vi "CSMSVMgr unload File.vi"(8 "error in (no error)":errorcluster, 10 "Path":path, 11 "CSM-Static-Variable-Manager in":refnum<class "CSM-Static-Variable-Manager.lvclass">) -> (0 "error out":errorcluster, 3 "CSM-Static-Variable-Manager out":refnum<class "CSM-Static-Variable-Manager.lvclass">)   [LabVIEW 2017, in "INI-Static-Variable-Support.lvlib" / "CSM-Static-Variable-Manager.lvclass"]
uses:
  CSM-Static-Variable-Manager.lvclass
  CSM-Static-Variable-Manager.lvclass/CSM-Static-Variable-Manager.ctl
  LabVIEW-Config/Config.ctl
  LabVIEW-Config/LineToken.ctl
  LabVIEW-Config/LabVIEW-Config.lvlib
  <userlib>/_NEVSTOP/Communicable State Machine(CSM)/Communicable State Machine.lvlib
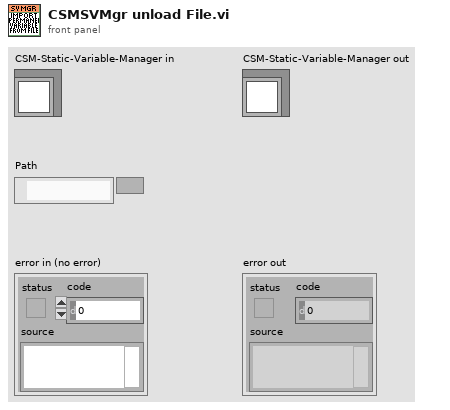
[diagram p1: front panel]
types:
  T1 = typedef "LabVIEW-Config.lvlib/Config.ctl" = cluster{"Path":path, "Lines":string[], "Tokens":T2[], "Modified?":bool}
  T2 = typedef "LabVIEW-Config.lvlib/LineToken.ctl" = enum8{"comment", "section", "key", "more"}
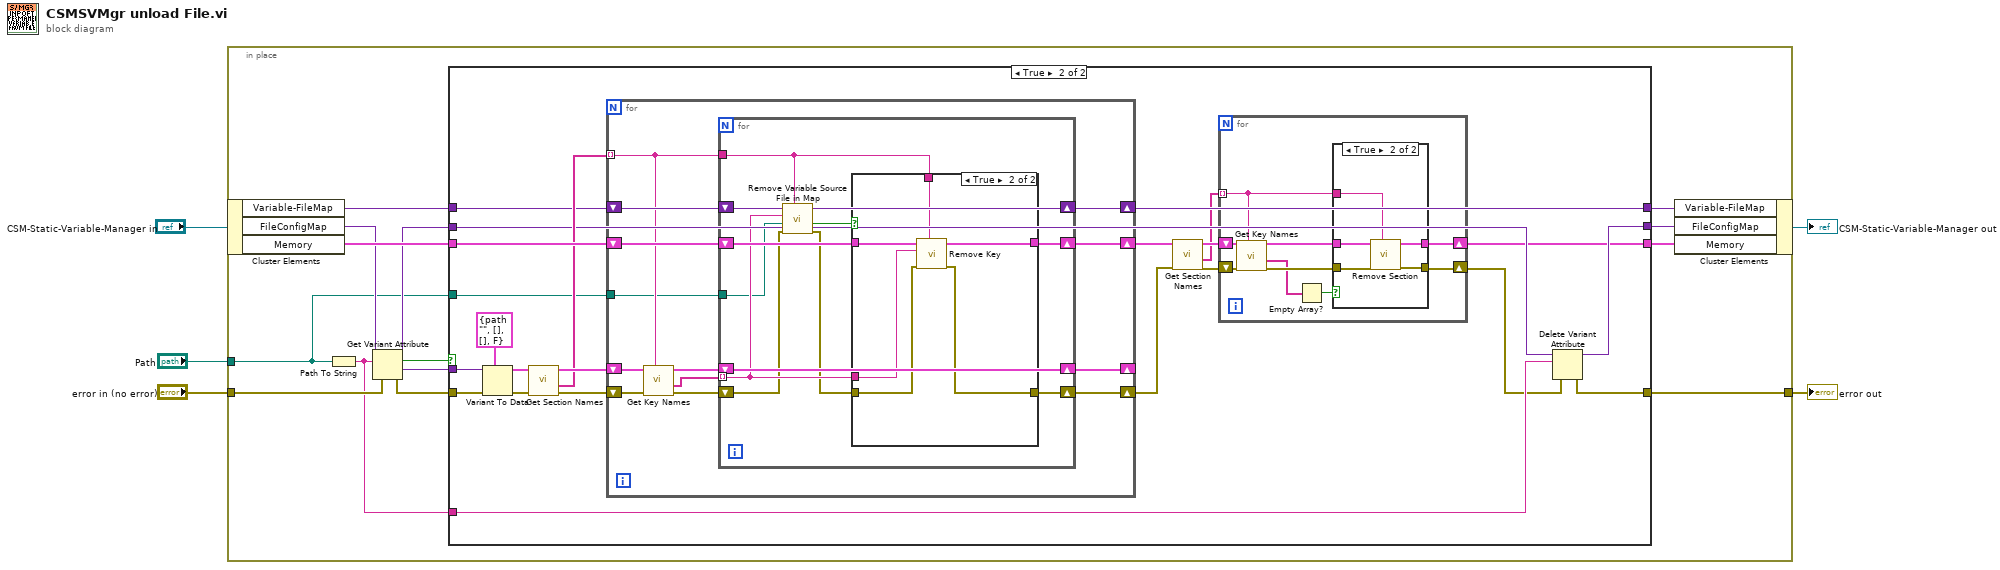
[diagram p0: block diagram]
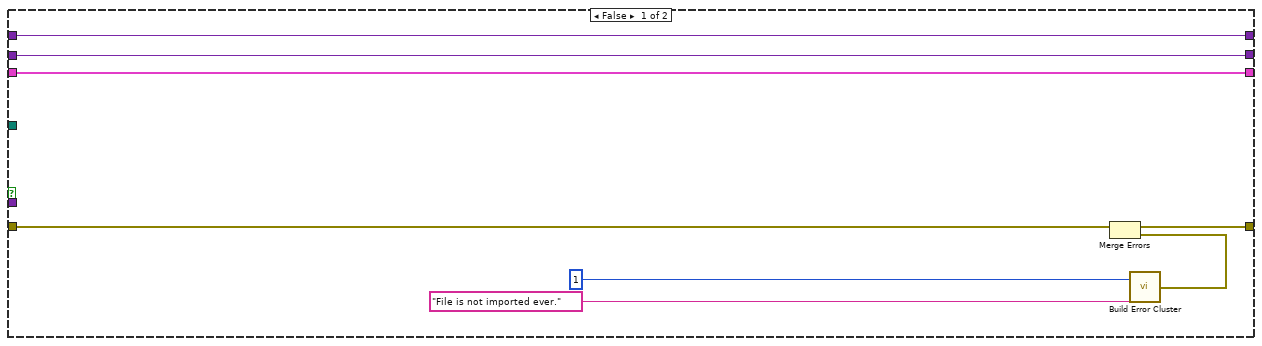
[diagram p2: hidden frame]
diagram:
  n1 = in-place {
    in-place-border: "error in (no error)" -> [w14]
    in-place-border: [w13] -> w2
    in-place-border: "Path" -> [w6]
    n2 = in-place-cluster #1("CSM-Static-Variable-Manager in") -> ("Variable-FileMap"=w9:variant, "FileConfigMap"=w17:variant, "Memory"=w19:T1)
    n3 = Path To String(path=w6) -> (string=w7:string)
    n4 = Get Variant Attribute(Variant=w17, name=w7, error in=w14) -> (duplicate Variant=w12:variant, found=w10:bool, value=w16:variant, error out=w15:errorcluster)  [unwired: 1 in]
    n5 = case shown="True" w10 {
      tunnel: w19 -> [w26 w50]
      tunnel: [w26 w31] -> w18
      tunnel: w16 -> [_ w49]
      tunnel: w15 -> [w25 w48]
      tunnel: [w24 w44] -> w13
      tunnel: w12 -> [w27 w39]
      tunnel: [w27 w43] -> w11
      tunnel: w9 -> [w20 w37]
      tunnel: [w20 w36] -> w8
      tunnel: w7 -> [_ w38]
      tunnel: w6 -> [_ w35]
      frame False {
        n6 = call <userlib>:"Build Error Cluster.vi"("String to Prepend to source (\"\")"="File is not imported ever." ("String to Prepend to source (\"\")"), "code"=1) -> ("error out"=w23:errorcluster)
        n7 = Merge Errors(w25, w23) -> (w24:errorcluster)
      }
      frame True {
        n8 = Variant To Data(error in=w48, type=T1 {"Path"=path "", "Lines"=[], "Tokens"=[], "Modified?"=FALSE}, Variant=w49) -> (data=w45:T1, error out=w47:errorcluster)
        n9 = call "Get Section Names.vi"("error in (no error)"=w47, "Config in"=w45) -> ("error out"=w41:errorcluster, "Section Names"=w40:string[], "Config out"=w42:T1)  [unwired: 7 in]
        n10 = for {
          shift-right: [w76] -> w32
          shift-left: w50 -> [w77]
          shift-right: [w75] -> w30
          shift-left: w41 -> [w73]
          tunnel: w40 -> [w69] mode=indexing
          shift-right: [w72] -> _
          shift-left: w42 -> [w74]
          shift-right: [w71] -> w36
          shift-left: w37 -> [w70]
          tunnel: w35 -> [w67]
          n11 = call "Get Key Names.vi"("Section Name"=w69, "error in (no error)"=w73, "Config in"=w74) -> ("error out"=w68:errorcluster, "Key Names"=w78:string[], "Config out"=w79:T1)  [unwired: 5 in, 1 out]
          n12 = for {
            tunnel: w69 -> [w85]
            tunnel: w78 -> [w84] mode=indexing
            shift-right: [w88] -> w75
            shift-left: w68 -> [w83]
            shift-right: [w91] -> w76
            shift-left: w77 -> [w90]
            shift-right: [w89] -> w72
            shift-left: w79 -> [w89]
            shift-right: [w86] -> w71
            shift-left: w70 -> [w87]
            tunnel: w67 -> [w81]
            n13 = call "Remove Variable Source File in Map.vi"("String"=w85, "error in (no error)"=w83, "dup path"=w81, "Content"=w84, "Variable-FileMap"=w87) -> ("error out"=w82:errorcluster, "No Source Any More?"=w80:bool, "Variant"=w86:variant)  [unwired: 4 in]
            n14 = case shown="True" w80 {
              tunnel: [w93 w99] -> w91
              tunnel: w90 -> [w93 w98]
              tunnel: [w92 w97] -> w88
              tunnel: w85 -> [_ w96]
              tunnel: w84 -> [_ w95]
              tunnel: w82 -> [w92 w94]
              frame False {
              }
              frame True {
                n15 = call "Remove Key.vi"("Section Name"=w96, "error in (no error)"=w94, "Key Name"=w95, "Config in"=w98) -> ("error out"=w97:errorcluster, "Config out"=w99:T1)  [unwired: 5 in, 1 out]
              }
            }
          }
        }
        n16 = call "Get Section Names.vi"("error in (no error)"=w30, "Config in"=w32) -> ("error out"=w33:errorcluster, "Section Names"=w28:string[], "Config out"=w34:T1)  [unwired: 7 in]
        n17 = for {
          shift-right: [w53] -> w31
          shift-left: w34 -> [w59]
          shift-right: [w52] -> w29
          shift-left: w33 -> [w56]
          tunnel: w28 -> [w51] mode=indexing
          n18 = call "Get Key Names.vi"("Section Name"=w51, "error in (no error)"=w56, "Config in"=w59) -> ("error out"=w57:errorcluster, "Key Names"=w55:string[], "Config out"=w58:T1)  [unwired: 5 in, 1 out]
          n19 = Empty Array?(array=w55) -> (empty?=w54:bool)
          n20 = case shown="True" w54 {
            tunnel: w58 -> [w61 w66]
            tunnel: w57 -> [w60 w65]
            tunnel: [w61 w64] -> w53
            tunnel: [w60 w63] -> w52
            tunnel: w51 -> [_ w62]
            frame False {
            }
            frame True {
              n21 = call "Remove Section.vi"("Section Name"=w62, "error in (no error)"=w65, "Config in"=w66) -> ("error out"=w63:errorcluster, "Config out"=w64:T1)  [unwired: 6 in, 1 out]
            }
          }
        }
        n22 = Delete Variant Attribute(4:w29, 6:w38, 7:w39) -> (0:w44:errorcluster, 3:w43:variant)  [unwired: 1 out]
      }
    }
    n23 = in-place-cluster #1("Variable-FileMap"=w8, "FileConfigMap"=w11, "Memory"=w18) -> (→"CSM-Static-Variable-Manager out":refnum<class "CSM-Static-Variable-Manager.lvclass">)
  }
  "error out" <- w2
